vi "Save OptiTrack Config.vi"(11 "Offset Array":dbl[](array[numeric])) -> (0 "error out":errorcluster)   [LabVIEW 2022 SP3]
uses:
  Anemometry/Anemometry Sub Vis/Globals/Constants_global.vi
  <vilib>/Utility/config.llb/Write Key (String).vi
  <vilib>/Utility/config.llb/NI_LVConfig.lvlib
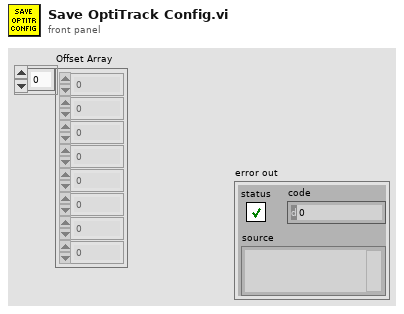
[diagram p1: front panel]
types:
  T1 = typedef "NI_LVConfig.lvlib/Config Data RefNum.ctl" = refnum<k1>
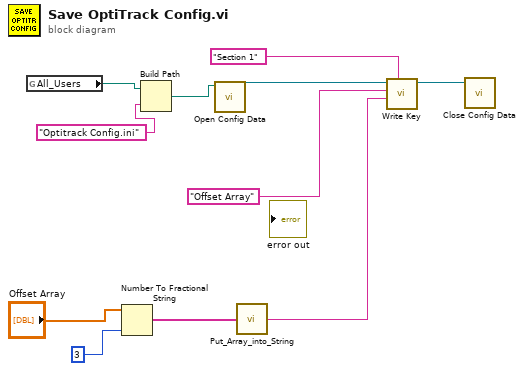
[diagram p0: block diagram]
diagram:
  n1 = global read "Constants_global.vi" "All_Users"() -> (w11:path)
  n2 = Number To Fractional String(number="Offset Array", precision (6)=i16 3) -> (F-format string=w6:string[])  [unwired: 2 in]
  n3 = Build Path(base path=w11, name or relative path="Optitrack Config.ini") -> (appended path=w9:path)
  n4 = call <vilib>:"Open Config Data.vi"("configuration file path"=w9) -> ("refnum"=w4:T1)  [unwired: 2 in, 8 out]
  n5 = call "Put_Array_into_String.vi"("String array"=w6) -> ("String Value"=w2:string)
  n6 = call-poly <vilib>:"Write Key.vi"("section"="Section 1", "value"=w2, "key"="Offset Array", "refnum"=w4) -> ("refnum out"=w1:T1)  [unwired: 5 in, 2 out]
  n7 = call <vilib>:"Close Config Data.vi"("refnum"=w1) -> ()  [unwired: 9 in, 2 out]
